vi "06.New_Evd.3_Ask.3.vi"() -> ()   [LabVIEW 2025]
panel:
  out "Array 2'":dbl[](array[knob]) scale=0.0..50.0
  in  "Array 3":dbl[](array[numeric])
  out "Array 1'":bool[][](array[boolean])
  in  "Array 1":bool[][](array[boolean])
  out "Path 2":path
  in  "Path":path
  in  "Waveform":waveform(dbl)
  out "Waveform Graph":waveform(dbl)(graph)
  out "String to Number":u32
  out "Number to String":string
  out "Integer":u32
  in  "Integer":i32
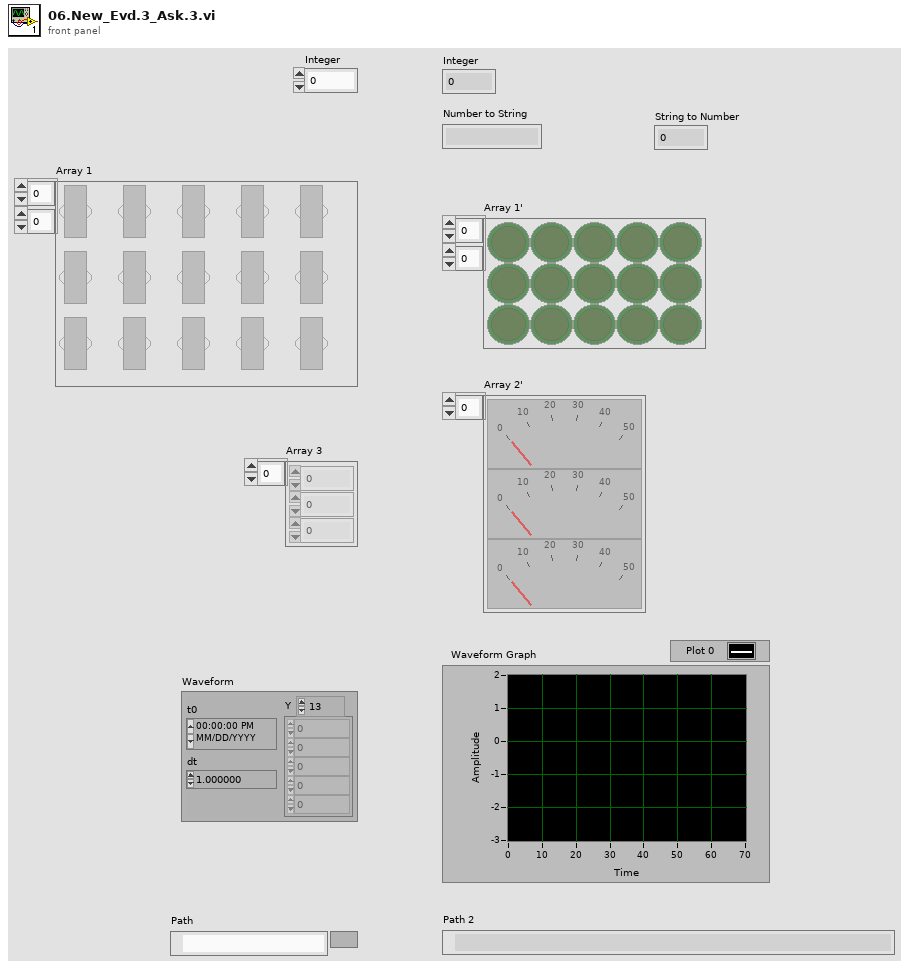
[diagram p1: front panel]
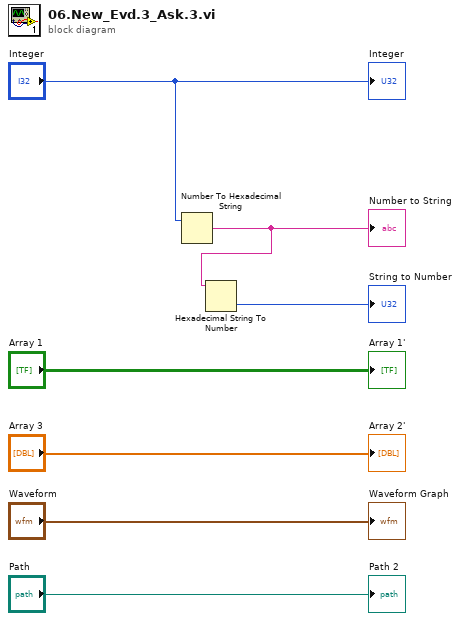
[diagram p0: block diagram]
diagram:
  n1 = Number To Hexadecimal String(2:"Integer") -> (0:w4:string)  [unwired: 1 in]
  "Number to String" <- w4
  n2 = Hexadecimal String To Number(string=w4) -> (number=→"String to Number":u32)  [unwired: 2 in, 1 out]
  "Integer" <- "Integer"
  "Waveform Graph" <- "Waveform"
  "Path 2" <- "Path"
  "Array 1'" <- "Array 1"
  "Array 2'" <- "Array 3"
